vi "CRYSet Default Configuration.vi"   [LabVIEW 2013]
doc: "Config File Reading/Writting\n\nPath \n ini File path\nRWFlag\n 0: no action\n 1: read\n 2: write"
uses:
  CRYMainGlobal.vi
  CRYStepSetup/CRYStepSetup Global.vi
  CRYProject/CRYProject Editor Global.vi
panel:
  # "Default Path cofigure setting"
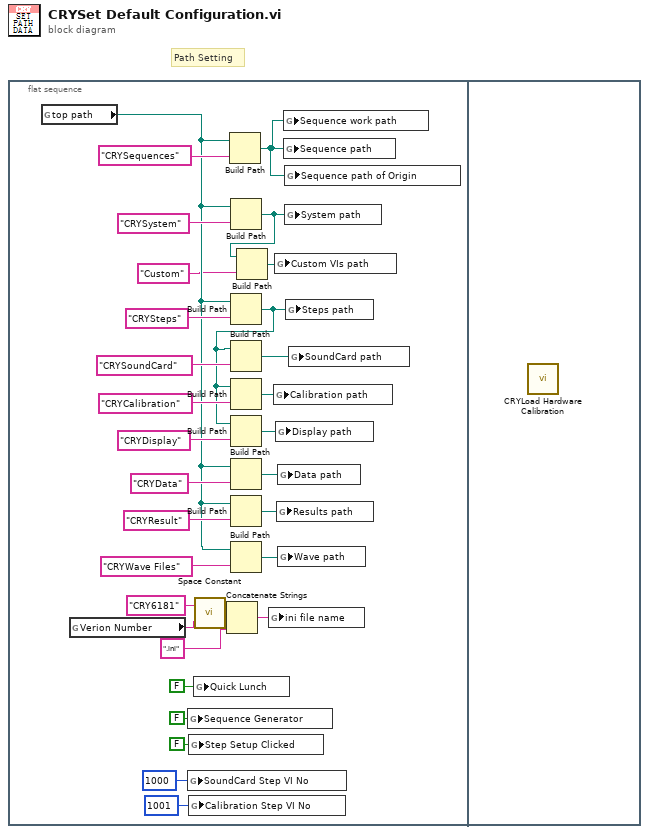
[diagram p0: block diagram]
diagram:
  # "Path Setting"
  n1 = flat-sequence {
    frame #0 {
      n2 = global read "CRYMainGlobal.vi" "top path"() -> (w4:path)
      n3 = global read "CRYMainGlobal.vi" "Verion Number"() -> (w8:string)
      n4 = global write "CRYMainGlobal.vi" "Sequence Generator"(FALSE ("Sequence Generator")) -> ()
      n5 = global write "CRYProject Editor Global.vi" "SoundCard Step VI No"(1000 ("Hardware Step VI No")) -> ()
      n6 = global write "CRYStepSetup Global.vi" "Step Setup Clicked"(FALSE ("Step Step Clicked")) -> ()
      n7 = global write "CRYProject Editor Global.vi" "Calibration Step VI No"(1001 ("Calibration Step VI No")) -> ()
      n8 = global write "CRYMainGlobal.vi" "Quick Lunch"(FALSE ("Quick Lunch")) -> ()
      n9 = call <vilib>:"Space Constant.vi"() -> ("String"=w7:string)
      n10 = Concatenate Strings("CRY6181" ("ini file name"), w7, w8, ".ini" ("ini file name")) -> (w6:string)
      n11 = Build Path(base path=w4, name or relative path="CRYSequences") -> (appended path=w10:path)
      n12 = Build Path(base path=w4, name or relative path="CRYSystem") -> (appended path=w2:path)
      n13 = Build Path(base path=w4, name or relative path="CRYSteps") -> (appended path=w18:path)
      n14 = Build Path(base path=w18, name or relative path="CRYSoundCard") -> (appended path=w20:path)
      n15 = Build Path(base path=w18, name or relative path="CRYCalibration") -> (appended path=w26:path)
      n16 = Build Path(base path=w18, name or relative path="CRYDisplay") -> (appended path=w21:path)
      n17 = Build Path(base path=w4, name or relative path="CRYData") -> (appended path=w23:path)
      n18 = Build Path(base path=w4, name or relative path="CRYResult") -> (appended path=w24:path)
      n19 = Build Path(base path=w4, name or relative path="CRYWave Files") -> (appended path=w17:path)
      n20 = Build Path(base path=w2, name or relative path="Custom") -> (appended path=w3:path)
      n21 = global write "CRYMainGlobal.vi" "ini file name"(w6) -> ()
      n22 = global write "CRYMainGlobal.vi" "Calibration path"(w26) -> ()
      n23 = global write "CRYMainGlobal.vi" "Custom VIs path"(w3) -> ()
      n24 = global write "CRYMainGlobal.vi" "Display path"(w21) -> ()
      n25 = global write "CRYMainGlobal.vi" "Results path"(w24) -> ()
      n26 = global write "CRYMainGlobal.vi" "Data path"(w23) -> ()
      n27 = global write "CRYMainGlobal.vi" "Wave path"(w17) -> ()
      n28 = global write "CRYMainGlobal.vi" "Sequence work path"(w10) -> ()
      n29 = global write "CRYMainGlobal.vi" "Sequence path"(w10) -> ()
      n30 = global write "CRYMainGlobal.vi" "Sequence path of Origin"(w10) -> ()
      n31 = global write "CRYMainGlobal.vi" "System path"(w2) -> ()
      n32 = global write "CRYMainGlobal.vi" "Steps path"(w18) -> ()
      n33 = global write "CRYMainGlobal.vi" "SoundCard path"(w20) -> ()
    }
    frame #1 {
      n34 = call "CRYLoad Hardware Calibration.vi"() -> ()  [unwired: 16 in]
    }
  }
